vi "Update Control when Color Range Changes from Dashboard Port.vi"(11 "Cluster in":refnum<vi>) -> ()   [LabVIEW 2023]
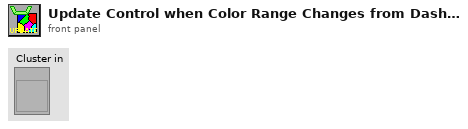
[diagram p1: front panel]
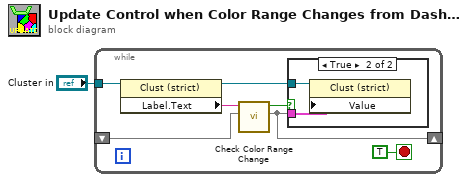
[diagram p0: block diagram]
diagram:
  n1 = while {
    tunnel: "Cluster in" -> [w4]
    shift-right: [w5] -> _
    shift-left: _ -> [w6]
    stop <- TRUE stop-if-true
    n2 = property class="Clust (strict)"(reference=w4) -> (reference out=w2:refnum<vi>, "Label.Text"=w3:string)  [unwired: 1 in, 1 out]
    n3 = call "Check Color Range Change.vi"(10:w6, "Name"=w3) -> (2:w5, "Changed"=w8:bool)  [unwired: 7 in, 1 out]
    n4 = case shown="True" w8 {
      tunnel: w5 -> [_ w10]
      tunnel: w2 -> [_ w9]
      frame False {
      }
      frame True {
        n5 = property on="Property Node" class="Clust (strict)"(reference=w9, "Value"=w10) -> ()  [unwired: 1 in, 2 out]
      }
    }
  }
